vi "Momentum Killer Demonstrator.vi"() -> ()   [LabVIEW 2011]
panel:
  out "Monitor":cluster{"Power Input":dbl, "Power Output":dbl}(graph)
  in  "Edge":bool=TRUE
  in  "Stop Delay (sec)":dbl=0.5
  in  "Reverse Power":dbl=-0.2
  in  "Reverse Time (sec)":dbl=0.3
  in  "Kill Control":bool
  out "Power Output":dbl
  in  "Power Input":dbl=0.5
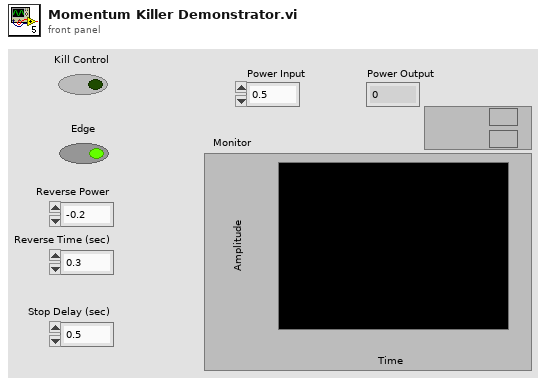
[diagram p1: front panel]
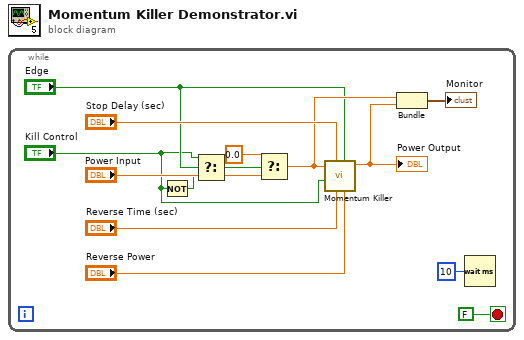
[diagram p0: block diagram]
diagram:
  n1 = while {
    stop <- FALSE stop-if-true
    n2 = Not(x="Kill Control") -> (.not. x?=w3:bool)
    n3 = Select(t="Kill Control", s="Edge", f=w3) -> (s? t:f=w2:bool)
    n4 = Select(t=0.0 ("f"), s=w2, f="Power Input") -> (s? t:f=w7:dbl)
    n5 = call "Momentum Killer.vi"("Reverse Power"="Reverse Power", "Edge"="Edge", "Reverse Time (sec)"="Reverse Time (sec)", "Stop Delay (sec)"="Stop Delay (sec)", "Kill Control"="Kill Control", "Power Input"=w7) -> ("Power Output"=w10:dbl)  [unwired: 5 in]
    "Power Output" <- w10
    n6 = Bundle("Power Input"=w7, "Power Output"=w10) -> (→"Monitor":cluster{"Power Input":dbl, "Power Output":dbl})  [unwired: 1 in]
    n7 = Wait (ms)(milliseconds to wait=u32 10) -> ()  [unwired: 1 out]
  }
